vi "ShowImage.vi"(2 "Color Table":T1(ring), 3 "Autoscale?":bool, 4 "Image":T2 {"Dialogs" format="%.0b"}) -> (0 "dimensions":cluster{"Witdh":i32, "Height":i32}, 1 "image":picture)   [LabVIEW 2014]
uses:
  QT_Image.ctl
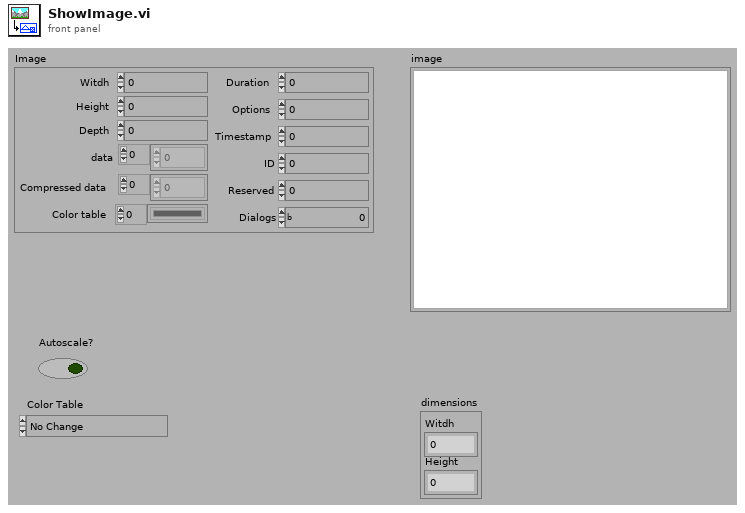
[diagram p1: front panel]
types:
  T1 = enum16{"No Change", "Apricot", "Carnation", "Ether", "Greyscale", "Greyscale-banded", "Hot Metal", "Lava Waves", "Mac", "Morning Glory", "Rainbow", "Rainbow-banded", "Rainbow-inverted", "Rainbow-striped", "Saturn", "Seismic", "Space"}
  T2 = typedef "QT_Image.ctl" = cluster{"Witdh":i32, "Height":i32, "Depth":i32, "data":u8[], "Compressed data":u8[], "Color table":u32[], "Duration":i32, "Options":i32, "Timestamp":i32, "ID":i32, "Reserved":i32, "Dialogs":u32}
  T3 = enum16{"Apricot", "Carnation", "Ether", "Greyscale", "Greyscale-banded", "Hot Metal", "Lava Waves", "Mac", "Morning Glory", "Rainbow", "Rainbow-banded", "Rainbow-inverted", "Rainbow-striped", "Saturn", "Seismic", "Space"}
  T4 = cluster{"left":i16, "top":i16, "right":i16, "bottom":i16}
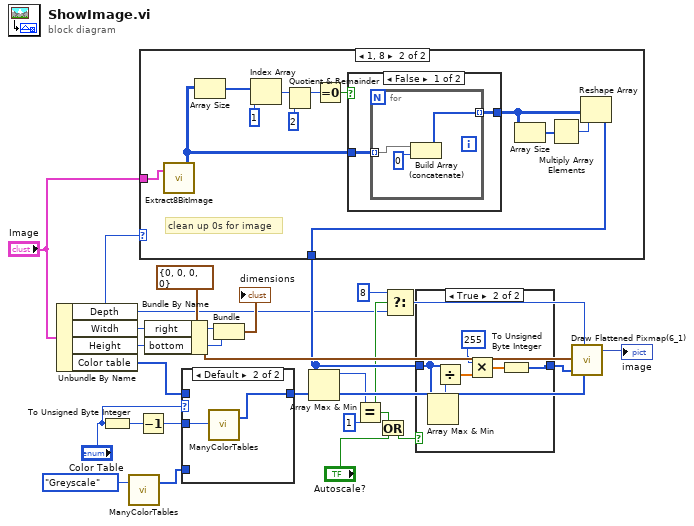
[diagram p0: block diagram]
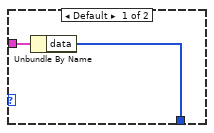
[diagram p2: hidden frame]
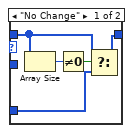
[diagram p5: hidden frame]
diagram:
  n1 = Unbundle By Name("Image") -> ("Depth"=w3:i32, "Witdh"=w22:i32, "Height"=w23:i32, "Color table"=w14:u32[])
  n2 = To Unsigned Byte Integer(number="Color Table") -> (unsigned 8bit integer=w17:u8)
  n3 = call "ManyColorTables.vi"("Color Table"=T3."Greyscale") -> ("Color Table Out"=w7:u32[])  [unwired: 2 out]
  n4 = Decrement(x=w17) -> (x-1=w16:u8)
  n5 = case shown="1, 8" w3 {
    tunnel: "Image" -> [w26 w36]
    tunnel: [w25 w35] -> w6
    frame Default {
      n6 = Unbundle By Name(w26) -> ("data"=w25:u8[])
    }
    frame 1, 8 {
      # "clean up 0s for image"
      n7 = call "Extract8BitImage.vi"("Image in"=w36) -> ("Intensity Graph"=w27:u8[][])  [unwired: 1 in, 1 out]
      n8 = Array Size(array=w27) -> (size(s)=w29:i32[])
      n9 = Index Array(array=w29, index=1) -> (element=w32:i32)
      n10 = Quotient & Remainder(x=w32, y=2) -> (x-y*floor(x/y)=w33:i32)  [unwired: 1 out]
      n11 = Equal To 0?(x=w33) -> (x = 0?=w30:bool)
      n12 = case shown="False" w30 {
        tunnel: [w40 w44] -> w28
        tunnel: w27 -> [w39 w44]
        frame False {
          n13 = for {
            tunnel: [w42] -> w40 mode=indexing
            tunnel: w39 -> [w41] mode=indexing
            n14 = Build Array (concatenate)(w41, u8 0) -> (w42:u8[])
          }
        }
        frame True {
        }
      }
      n15 = Array Size(array=w28) -> (size(s)=w37:i32[])
      n16 = Multiply Array Elements(1:w37) -> (0:w38:i32)
      n17 = Reshape Array(w28, w38) -> (w35:u8[])
    }
  }
  n18 = Bundle By Name(cluster=T4 {"left"=0, "top"=0, "right"=0, "bottom"=0} ("rect"), "right"=w22, "bottom"=w23) -> (w20:T4)
  n19 = case shown="Default" "Color Table" {
    tunnel: w16 -> [_ w51]
    tunnel: [w45 w50] -> w15
    tunnel: w14 -> [w47 _]
    tunnel: w7 -> [w46 _]
    frame "No Change" {
      n20 = Array Size(array=w47) -> (size(s)=w49:i32)
      n21 = Not Equal To 0?(x=w49) -> (x != 0?=w48:bool)
      n22 = Select(t=w47, s=w48, f=w46) -> (s? t:f=w45:u32[])
    }
    frame Default {
      n23 = call "ManyColorTables.vi"("Color Table"=w51) -> ("Color Table Out"=w50:u32[])  [unwired: 2 out]
    }
  }
  n24 = Bundle("Witdh"=w22, "Height"=w23) -> (→"dimensions":cluster{"Witdh":i32, "Height":i32})  [unwired: 1 out]
  n25 = Array Max & Min(array=w6) -> (max value=w5:u8)  [unwired: 3 out]
  n26 = Equal?(x=w5, y=u8 1) -> (x = y?=w4:bool)
  n27 = Or(x=w4, y="Autoscale?") -> (x .or. y?=w9:bool)
  n28 = Select(t=8, s=w4, f=w3) -> (s? t:f=w2:i32)
  n29 = case shown="True" w9 {
    tunnel: [w52 w53] -> w13
    tunnel: w6 -> [w52 w58]
    frame False {
    }
    frame True {
      n30 = Array Max & Min(array=w58) -> (max value=w57:u8)  [unwired: 3 out]
      n31 = Divide(x=w58, y=w57) -> (x/y=w56:dbl[])
      n32 = Multiply(x=i16 255 ("left"), y=w56) -> (x*y=w54:dbl[])
      n33 = To Unsigned Byte Integer(number=w54) -> (unsigned 8bit integer=w53:u8[])
    }
  }
  n34 = call <vilib>:"Draw Flattened Pixmap(6_1).vi"("bit depth(8)"=w2, "rect"=w20, "flattened pixmap data"=w13, "color table"=w15) -> ("new picture"=→"image":picture)  [unwired: 1 in, 4 out]
